vi "examen2.vi"() -> ()   [LabVIEW 2019]
panel:
  in  "# dulce":dbl
  in  "#bebida fria":dbl
  in  "#cafe":dbl
  in  "# snack":dbl
  in  "stop":bool
  in  "Tab Control":enum32{"Page 1", "Page 2"}(tab)
  in  "dulce":bool
  in  "bebida fria":bool
  in  "cafe":bool
  in  "snack":bool
  out "producto":bool
  out "agotado":string="Articulo agotado"
  out "Cambio":dbl
  out "cambio":bool
  out "agotadoled":bool
  in  "Monedas":cluster{"moneda 10":bool, "moneda 20":bool}
  out "Dinero ingresado":dbl
  in  "comprar":bool
  in  "Cancelar":bool
  in  "reset":bool
  # "1. Seleccione su producto\n2. Ingrese sus monedas\n3. Oprima el boton de comprar\n4. Recoja su producto\n5. Recoja su cambio"
  # "30$"
  # "40$"
  # "40$"
  # "30$"
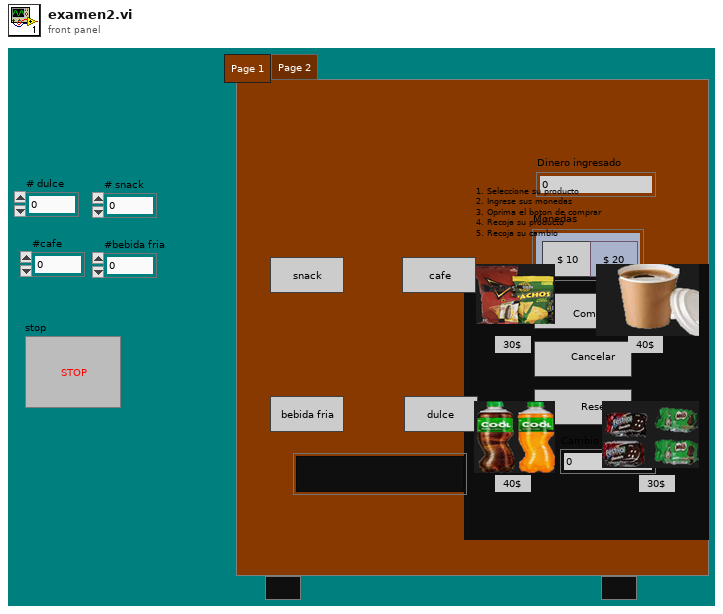
[diagram p1: front panel]
types:
  T1 = enum16{"inicio", "snack", "comprar s", "cambio s", "cafe", "comprar c", "cambio c", "bebida fria", "comprar bf", "cambio bf", "dulce", "comprar d", "cambio d", "reinicio", "cancelar"}
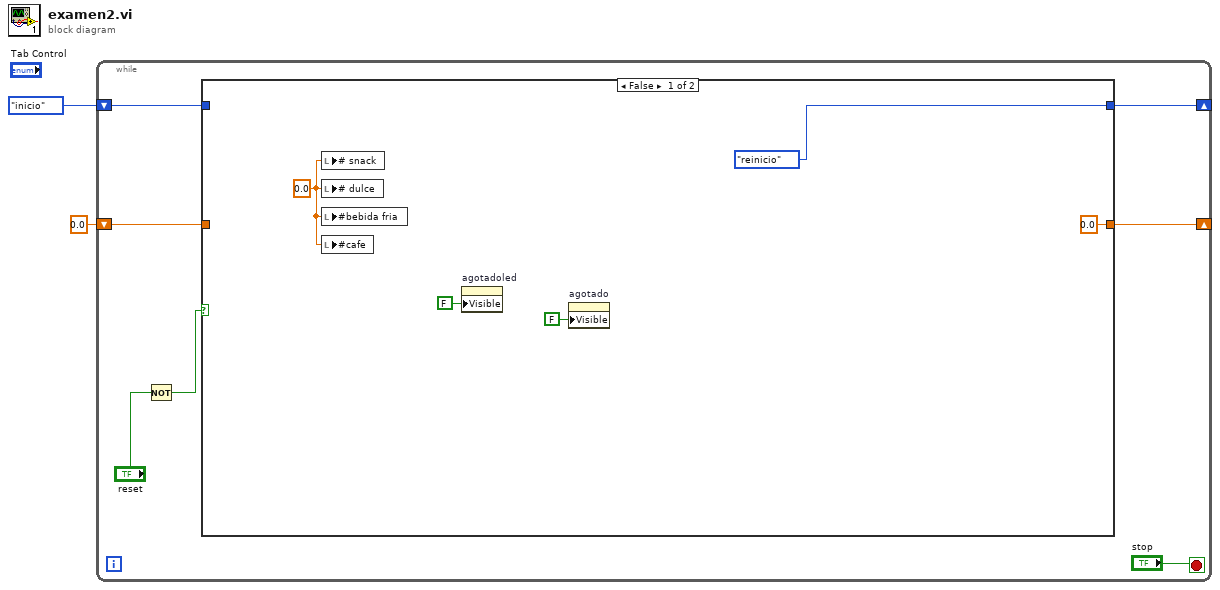
[diagram p0: block diagram]
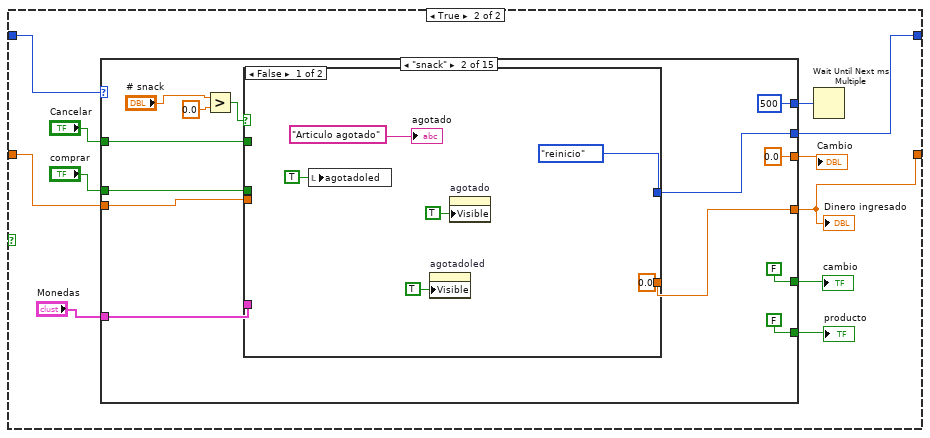
[diagram p2: hidden frame]
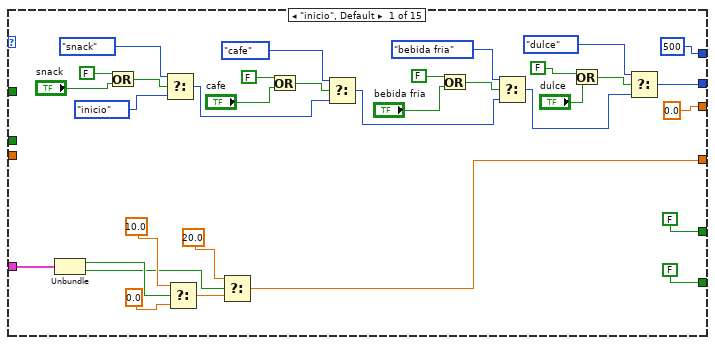
[diagram p3: hidden frame]
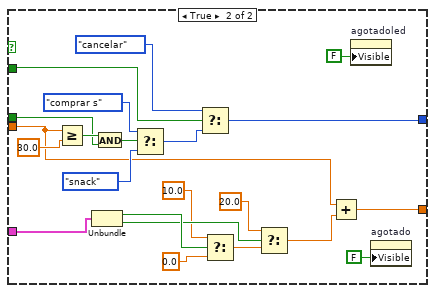
[diagram p4: hidden frame]
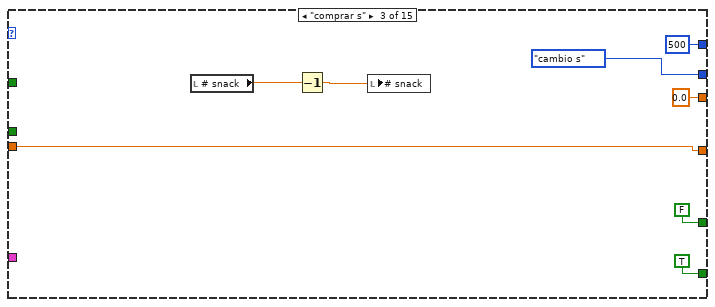
[diagram p5: hidden frame]
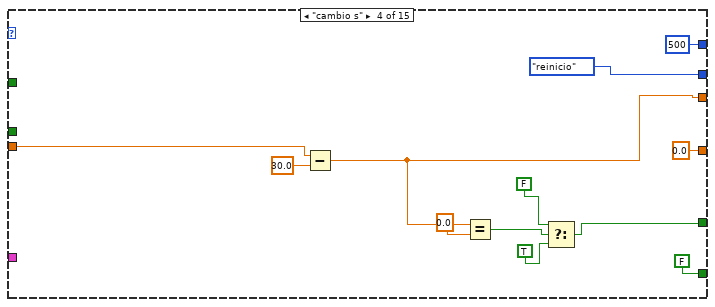
[diagram p6: hidden frame]
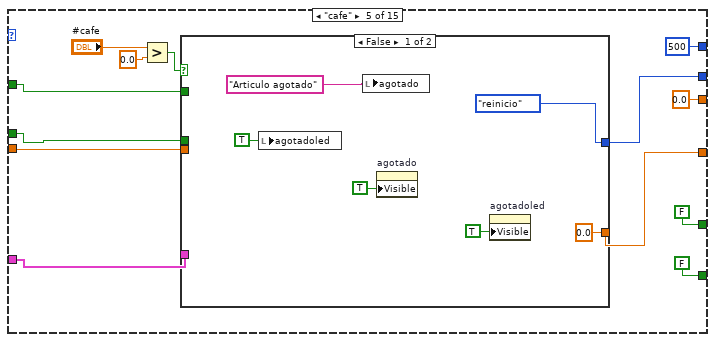
[diagram p7: hidden frame]
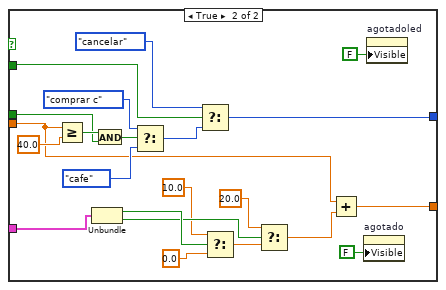
[diagram p8: hidden frame]
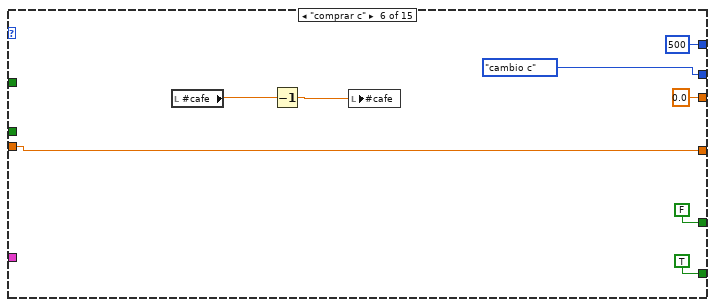
[diagram p9: hidden frame]
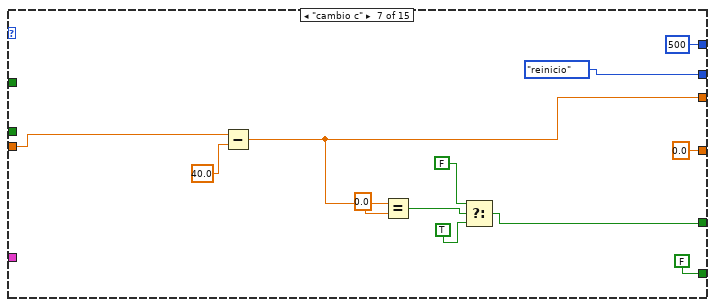
[diagram p10: hidden frame]
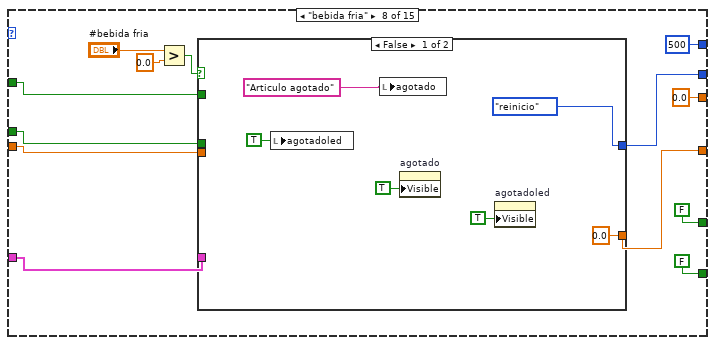
[diagram p11: hidden frame]
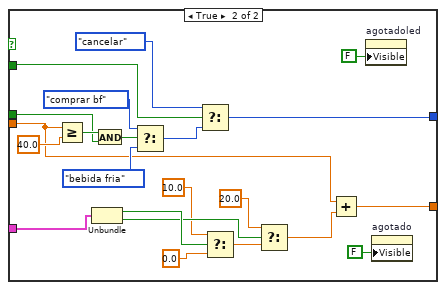
[diagram p12: hidden frame]
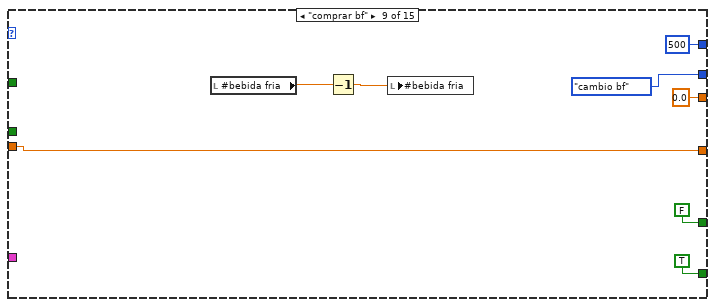
[diagram p13: hidden frame]
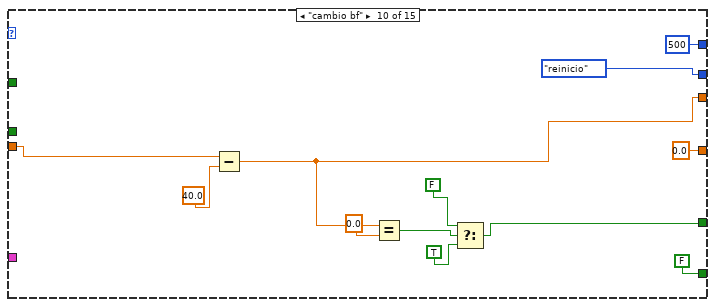
[diagram p14: hidden frame]
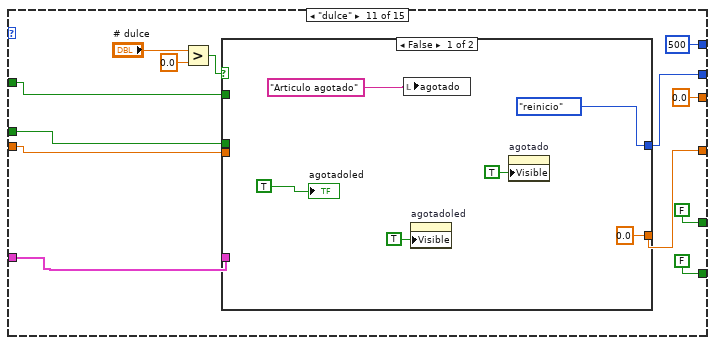
[diagram p15: hidden frame]
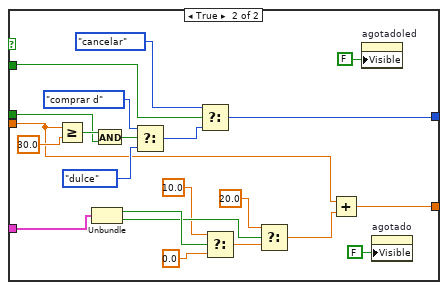
[diagram p16: hidden frame]
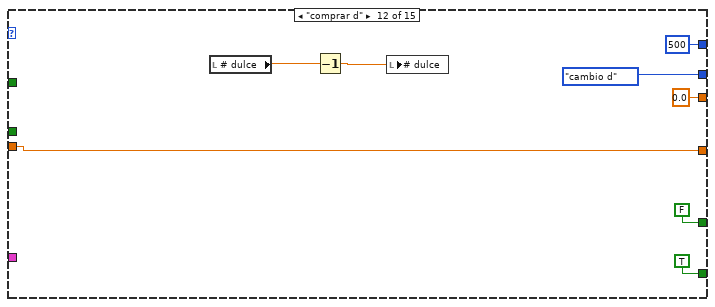
[diagram p17: hidden frame]
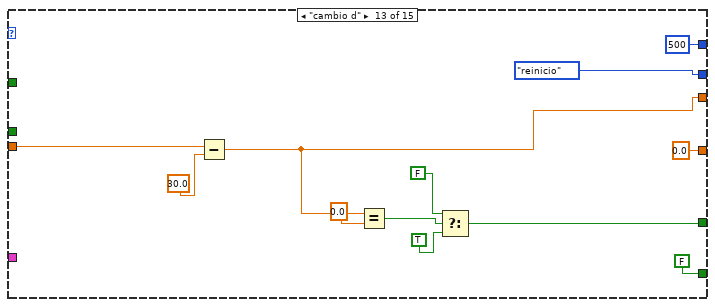
[diagram p18: hidden frame]
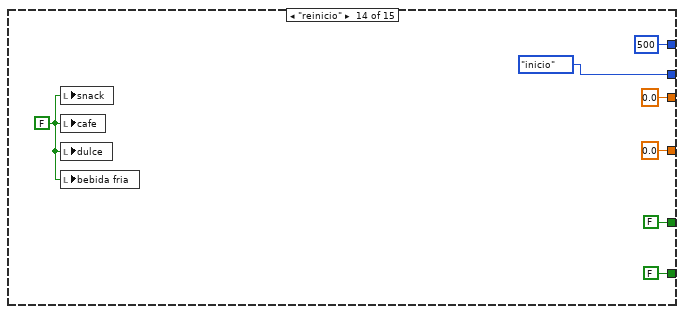
[diagram p19: hidden frame]
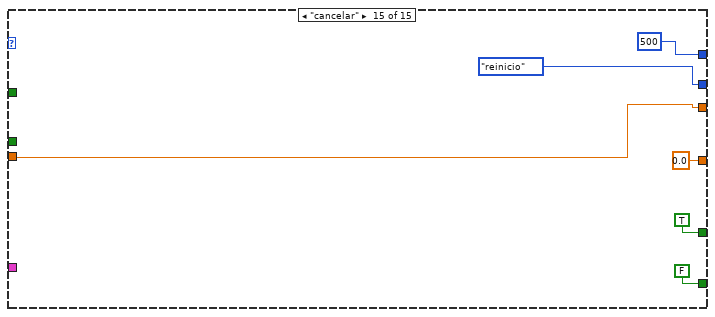
[diagram p20: hidden frame]
diagram:
  n1 = while {
    shift-right: [w8] -> _
    shift-left: T1."inicio" -> [w9]
    shift-right: [w7] -> _
    shift-left: 0.0 ("f") -> [w6]
    stop <- "stop" stop-if-true
    n2 = Not(x="reset") -> (.not. x?=w3:bool)
    n3 = case shown="False" w3 {
      tunnel: w9 -> [_ w25]
      tunnel: [T1."reinicio" w23] -> w8
      tunnel: [0.0 ("f") w18] -> w7
      tunnel: w6 -> [_ w17]
      frame False {
        w12 = 0.0
        n4 = local write "# snack"(w12) -> ()
        n5 = local write "# dulce"(w12) -> ()
        n6 = local write "#bebida fria"(w12) -> ()
        n7 = local write "#cafe"(w12) -> ()
        n8 = property on="agotadoled" class="Bool (strict)"("Visible"=FALSE) -> ()  [unwired: 2 in, 2 out]
        n9 = property on="agotado" class="Str"("Visible"=FALSE) -> ()  [unwired: 2 in, 2 out]
      }
      frame True {
        n10 = case shown="\"snack\"" w25 {
          tunnel: [500 500 500 500 500 500 500 500 500 500 500 500 500 500 500] -> w24
          tunnel: [w37 w64 T1."cambio s" T1."reinicio" w125 T1."cambio c" T1."reinicio" w186 T1."cambio bf" T1."reinicio" w246 T1."cambio d" T1."reinicio" T1."inicio" T1."reinicio"] -> w23
          tunnel: [0.0 0.0 0.0 w116 0.0 0.0 w171 0.0 0.0 w234 0.0 0.0 w294 0.0 w313] -> w22
          tunnel: "Monedas" -> [w35 w66 _ _ w126 _ _ w187 _ _ w251 _ _ _ _]
          tunnel: [w28 w65 w104 0.0 ("f") w124 w168 0.0 ("f") w183 w226 0.0 ("f") w245 w287 0.0 ("f") 0.0 ("f") 0.0 ("f")] -> w18
          tunnel: [FALSE FALSE TRUE FALSE FALSE TRUE FALSE FALSE TRUE FALSE FALSE TRUE FALSE FALSE FALSE] -> w20
          tunnel: [FALSE FALSE FALSE w112 FALSE FALSE w173 FALSE FALSE w232 FALSE FALSE w293 FALSE TRUE] -> w19
          tunnel: w17 -> [_ w69 w104 w119 w127 w168 w169 w188 w226 w230 w250 w287 w291 _ w313]
          tunnel: "comprar" -> [_ w68 _ _ w128 _ _ w189 _ _ w249 _ _ _ _]
          tunnel: "Cancelar" -> [_ w67 _ _ w129 _ _ w190 _ _ w248 _ _ _ _]
          frame "inicio", Default {
            n11 = Unbundle(w35) -> ("moneda 10"=w34:bool, "moneda 20"=w30:bool)
            n12 = Or(x=FALSE, y="snack") -> (x .or. y?=w56:bool)
            n13 = Select(t=T1."snack", s=w56, f=T1."inicio") -> (s? t:f=w49:T1)
            n14 = Select(t=10.0, s=w34, f=0.0) -> (s? t:f=w31:dbl)
            n15 = Select(t=20.0, s=w30, f=w31) -> (s? t:f=w28:dbl)
            n16 = Or(x=FALSE, y="cafe") -> (x .or. y?=w52:bool)
            n17 = Select(t=T1."cafe", s=w52, f=w49) -> (s? t:f=w44:T1)
            n18 = Or(x=FALSE, y="bebida fria") -> (x .or. y?=w47:bool)
            n19 = Select(t=T1."bebida fria", s=w47, f=w44) -> (s? t:f=w39:T1)
            n20 = Or(x=FALSE, y="dulce") -> (x .or. y?=w42:bool)
            n21 = Select(t=T1."dulce", s=w42, f=w39) -> (s? t:f=w37:T1)
          }
          frame "snack" {
            n22 = Greater?(x="# snack", y=0.0) -> (0:w70:bool)
            n23 = case shown="False" w70 {
              tunnel: w69 -> [_ w83]
              tunnel: w68 -> [_ w94]
              tunnel: w67 -> [_ w81]
              tunnel: w66 -> [_ w85]
              tunnel: [0.0 w82] -> w65
              tunnel: [T1."reinicio" w80] -> w64
              frame False {
                n24 = local write "agotadoled"(TRUE ("agotadoled")) -> ()
                n25 = property on="agotadoled" class="Bool (strict)"("Visible"=TRUE) -> ()  [unwired: 2 in, 2 out]
                n26 = property on="agotado" class="Str"("Visible"=TRUE) -> ()  [unwired: 2 in, 2 out]
                "agotado" <- "Articulo agotado"
              }
              frame True {
                n27 = Greater Or Equal?(x=w83, y=30.0) -> (x >= y?=w98:bool)
                n28 = Unbundle(w85) -> ("moneda 10"=w91:bool, "moneda 20"=w89:bool)
                n29 = And(x=w98, y=w94) -> (x .and. y?=w99:bool)
                n30 = Select(t=T1."comprar s", s=w99, f=T1."snack") -> (s? t:f=w93:T1)
                n31 = Select(t=T1."cancelar", s=w81, f=w93) -> (s? t:f=w80:T1)
                n32 = Select(t=10.0, s=w91, f=0.0) -> (s? t:f=w90:dbl)
                n33 = Select(t=20.0, s=w89, f=w90) -> (s? t:f=w84:dbl)
                n34 = Add(x=w83, y=w84) -> (x+y=w82:dbl)
                n35 = property on="agotadoled" class="Bool (strict)"("Visible"=FALSE) -> ()  [unwired: 2 in, 2 out]
                n36 = property on="agotado" class="Str"("Visible"=FALSE) -> ()  [unwired: 2 in, 2 out]
              }
            }
          }
          frame "comprar s" {
            n37 = local read "# snack"() -> (w101:dbl)
            n38 = Decrement(x=w101) -> (x-1=w100:dbl)
            n39 = local write "# snack"(w100) -> ()
          }
          frame "cambio s" {
            n40 = Subtract(x=w119, y=30.0) -> (x-y=w116:dbl)
            n41 = Equal?(x=w116, y=0.0) -> (x = y?=w114:bool)
            n42 = Select(t=FALSE, s=w114, f=TRUE) -> (s? t:f=w112:bool)
          }
          frame "cafe" {
            n43 = Greater?(x="#cafe", y=0.0) -> (0:w130:bool)
            n44 = case shown="False" w130 {
              tunnel: w127 -> [_ w144]
              tunnel: w128 -> [_ w155]
              tunnel: w129 -> [_ w142]
              tunnel: w126 -> [_ w146]
              tunnel: [0.0 w143] -> w124
              tunnel: [T1."reinicio" w141] -> w125
              frame False {
                n45 = local write "agotadoled"(TRUE ("agotadoled")) -> ()
                n46 = local write "agotado"("Articulo agotado") -> ()
                n47 = property on="agotado" class="Str"("Visible"=TRUE) -> ()  [unwired: 2 in, 2 out]
                n48 = property on="agotadoled" class="Bool (strict)"("Visible"=TRUE) -> ()  [unwired: 2 in, 2 out]
              }
              frame True {
                n49 = Greater Or Equal?(x=w144, y=40.0) -> (x >= y?=w159:bool)
                n50 = Unbundle(w146) -> ("moneda 10"=w152:bool, "moneda 20"=w150:bool)
                n51 = And(x=w159, y=w155) -> (x .and. y?=w160:bool)
                n52 = Select(t=T1."comprar c", s=w160, f=T1."cafe") -> (s? t:f=w154:T1)
                n53 = Select(t=T1."cancelar", s=w142, f=w154) -> (s? t:f=w141:T1)
                n54 = Select(t=10.0, s=w152, f=0.0) -> (s? t:f=w151:dbl)
                n55 = Select(t=20.0, s=w150, f=w151) -> (s? t:f=w145:dbl)
                n56 = Add(x=w144, y=w145) -> (x+y=w143:dbl)
                n57 = property on="agotado" class="Str"("Visible"=FALSE) -> ()  [unwired: 2 in, 2 out]
                n58 = property on="agotadoled" class="Bool (strict)"("Visible"=FALSE) -> ()  [unwired: 2 in, 2 out]
              }
            }
          }
          frame "comprar c" {
            n59 = local read "#cafe"() -> (w162:dbl)
            n60 = Decrement(x=w162) -> (x-1=w161:dbl)
            n61 = local write "#cafe"(w161) -> ()
          }
          frame "cambio c" {
            n62 = Subtract(x=w169, y=40.0) -> (x-y=w171:dbl)
            n63 = Equal?(x=w171, y=0.0) -> (x = y?=w176:bool)
            n64 = Select(t=FALSE, s=w176, f=TRUE) -> (s? t:f=w173:bool)
          }
          frame "bebida fria" {
            n65 = Greater?(x="#bebida fria", y=0.0) -> (0:w191:bool)
            n66 = case shown="False" w191 {
              tunnel: w188 -> [_ w205]
              tunnel: w189 -> [_ w216]
              tunnel: w190 -> [_ w203]
              tunnel: w187 -> [_ w207]
              tunnel: [0.0 w204] -> w183
              tunnel: [T1."reinicio" w202] -> w186
              frame False {
                n67 = local write "agotadoled"(TRUE ("agotadoled")) -> ()
                n68 = local write "agotado"("Articulo agotado") -> ()
                n69 = property on="agotado" class="Str"("Visible"=TRUE) -> ()  [unwired: 2 in, 2 out]
                n70 = property on="agotadoled" class="Bool (strict)"("Visible"=TRUE) -> ()  [unwired: 2 in, 2 out]
              }
              frame True {
                n71 = Greater Or Equal?(x=w205, y=40.0) -> (x >= y?=w220:bool)
                n72 = Unbundle(w207) -> ("moneda 10"=w213:bool, "moneda 20"=w211:bool)
                n73 = And(x=w220, y=w216) -> (x .and. y?=w221:bool)
                n74 = Select(t=T1."comprar bf", s=w221, f=T1."bebida fria") -> (s? t:f=w215:T1)
                n75 = Select(t=T1."cancelar", s=w203, f=w215) -> (s? t:f=w202:T1)
                n76 = Select(t=10.0, s=w213, f=0.0) -> (s? t:f=w212:dbl)
                n77 = Select(t=20.0, s=w211, f=w212) -> (s? t:f=w206:dbl)
                n78 = Add(x=w205, y=w206) -> (x+y=w204:dbl)
                n79 = property on="agotadoled" class="Bool (strict)"("Visible"=FALSE) -> ()  [unwired: 2 in, 2 out]
                n80 = property on="agotado" class="Str"("Visible"=FALSE) -> ()  [unwired: 2 in, 2 out]
              }
            }
          }
          frame "comprar bf" {
            n81 = local read "#bebida fria"() -> (w223:dbl)
            n82 = Decrement(x=w223) -> (x-1=w222:dbl)
            n83 = local write "#bebida fria"(w222) -> ()
          }
          frame "cambio bf" {
            n84 = Subtract(x=w230, y=40.0) -> (x-y=w234:dbl)
            n85 = Equal?(x=w234, y=0.0) -> (x = y?=w237:bool)
            n86 = Select(t=FALSE, s=w237, f=TRUE) -> (s? t:f=w232:bool)
          }
          frame "dulce" {
            n87 = Greater?(x="# dulce", y=0.0) -> (0:w253:bool)
            n88 = case shown="False" w253 {
              tunnel: w250 -> [_ w266]
              tunnel: w249 -> [_ w277]
              tunnel: w248 -> [_ w264]
              tunnel: w251 -> [_ w268]
              tunnel: [0.0 w265] -> w245
              tunnel: [T1."reinicio" w263] -> w246
              frame False {
                n89 = local write "agotado"("Articulo agotado") -> ()
                n90 = property on="agotadoled" class="Bool (strict)"("Visible"=TRUE) -> ()  [unwired: 2 in, 2 out]
                n91 = property on="agotado" class="Str"("Visible"=TRUE) -> ()  [unwired: 2 in, 2 out]
                "agotadoled" <- TRUE
              }
              frame True {
                n92 = Greater Or Equal?(x=w266, y=30.0) -> (x >= y?=w281:bool)
                n93 = Unbundle(w268) -> ("moneda 10"=w274:bool, "moneda 20"=w272:bool)
                n94 = And(x=w281, y=w277) -> (x .and. y?=w282:bool)
                n95 = Select(t=T1."comprar d", s=w282, f=T1."dulce") -> (s? t:f=w276:T1)
                n96 = Select(t=T1."cancelar", s=w264, f=w276) -> (s? t:f=w263:T1)
                n97 = Select(t=10.0, s=w274, f=0.0) -> (s? t:f=w273:dbl)
                n98 = Select(t=20.0, s=w272, f=w273) -> (s? t:f=w267:dbl)
                n99 = Add(x=w266, y=w267) -> (x+y=w265:dbl)
                n100 = property on="agotadoled" class="Bool (strict)"("Visible"=FALSE) -> ()  [unwired: 2 in, 2 out]
                n101 = property on="agotado" class="Str"("Visible"=FALSE) -> ()  [unwired: 2 in, 2 out]
              }
            }
          }
          frame "comprar d" {
            n102 = local read "# dulce"() -> (w284:dbl)
            n103 = Decrement(x=w284) -> (x-1=w283:dbl)
            n104 = local write "# dulce"(w283) -> ()
          }
          frame "cambio d" {
            n105 = Subtract(x=w291, y=30.0) -> (x-y=w294:dbl)
            n106 = Equal?(x=w294, y=0.0) -> (x = y?=w297:bool)
            n107 = Select(t=FALSE, s=w297, f=TRUE) -> (s? t:f=w293:bool)
          }
          frame "reinicio" {
            w303 = FALSE
            n108 = local write "snack"(w303) -> ()
            n109 = local write "cafe"(w303) -> ()
            n110 = local write "dulce"(w303) -> ()
            n111 = local write "bebida fria"(w303) -> ()
          }
          frame "cancelar" {
          }
        }
        "Cambio" <- w22
        "Dinero ingresado" <- w18
        "cambio" <- w19
        "producto" <- w20
        n112 = Wait Until Next ms Multiple(millisecond multiple=w24) -> ()  [unwired: 1 out]
      }
    }
  }
